vi "Error To Console.vi"(8 "error in (no error)":errorcluster, 11 "Add Text to Message":string) -> ()   [LabVIEW 2017, in "Shared Variables CD 2.0 Engine.lvlib"]
uses:
  Shared Variables CD 2.0 Engine.lvlib
  <vilib>/NI Veristand/Custom Device Tools/Custom Device Utility Library/Custom Device Utility Library.lvlib
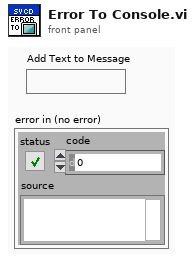
[diagram p1: front panel]
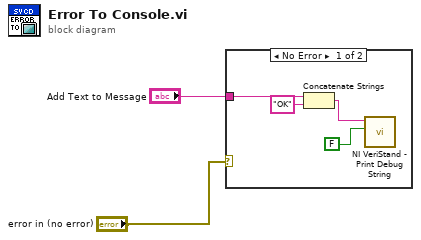
[diagram p0: block diagram]
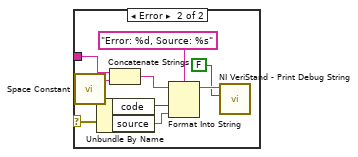
[diagram p2: hidden frame]
diagram:
  n1 = case shown="No Error" "error in (no error)" {
    selector: "error in (no error)" -> [_ w15]
    tunnel: "Add Text to Message" -> [w6 w9]
    frame No Error {
      n2 = Concatenate Strings(w6, "OK" ("string")) -> (w4:string)
      n3 = call <vilib>:"NI VeriStand - Print Debug String.vi"("Add to log file? (T)"=FALSE, "Message"=w4) -> ()  [unwired: 9 in, 1 out]
    }
    frame Error {
      n4 = call <vilib>:"Space Constant.vi"() -> ("String"=w7:string)
      n5 = Unbundle By Name(w15) -> ("code"=w14:i32, "source"=w13:string)
      n6 = Concatenate Strings(w9, w7) -> (w8:string)
      n7 = Format Into String(format string="Error: %d, Source: %s", initial string=w8, w14, w13) -> (resulting string=w12:string)  [unwired: 1 in, 1 out]
      n8 = call <vilib>:"NI VeriStand - Print Debug String.vi"("Add to log file? (T)"=FALSE, "Message"=w12) -> ()  [unwired: 9 in, 1 out]
    }
  }
